vi "second order system.vi"(8 "delta t":dbl=0.01 format="%.2f", 9 "damp":dbl=1.0 format="%.2f", 10 "omega n":dbl=1.0 format="%.2f", 11 "command":dbl format="%.2f") -> (2 "response":dbl(graph)=-42.44427756719487)   [LabVIEW 2016]
doc: "This subVI mimics a second order system."
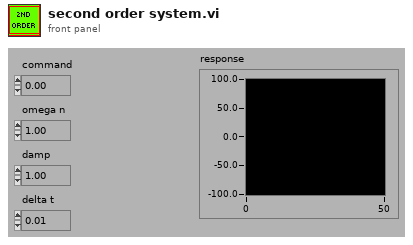
[diagram p1: front panel]
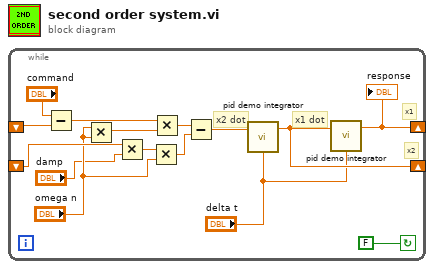
[diagram p0: block diagram]
diagram:
  n1 = while {
    shift-left: _ -> [w14]
    shift-right: [w13] -> _
    shift-left: _ -> [w11]
    shift-right: [w2] -> _
    stop <- FALSE continue-if-true
    # "x2 dot"
    # "x1 dot"
    # "x2"
    # "x1"
    n2 = Subtract(x="command", y=w11) -> (x-y=w10:dbl)
    n3 = Multiply(x="omega n", y="omega n") -> (x*y=w9:dbl)
    n4 = Multiply(x=w14, y="damp") -> (x*y=w8:dbl)
    n5 = Multiply(x=w8, y="omega n") -> (x*y=w7:dbl)
    n6 = Multiply(x=w10, y=w9) -> (x*y=w5:dbl)
    n7 = Subtract(x=w5, y=w7) -> (x-y=w15:dbl)
    n8 = call "pid demo integrator.vi"("delta t"="delta t", "input"=w15) -> ("output"=w13:dbl)  [unwired: 3 in]
    n9 = call "pid demo integrator.vi"("delta t"="delta t", "input"=w13) -> ("output"=w2:dbl)  [unwired: 3 in]
    "response" <- w2
  }
